vi "ReadFromTxt.vi"(11 "path to PNG file":path) -> (2 "image data":T1)   [LabVIEW 2017]
uses:
  <vilib>/picture/picture.llb/imagedata.ctl
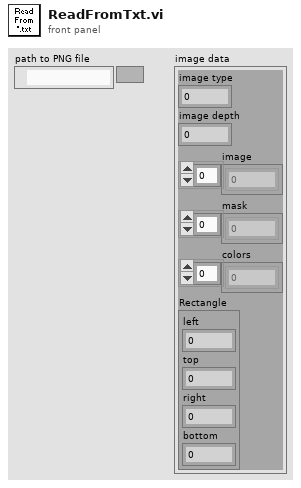
[diagram p1: front panel]
types:
  T1 = typedef "imagedata.ctl" = cluster{"image type":i32, "image depth":i32, "image":u8[], "mask":u8[], "colors":u32[], "Rectangle":cluster{"left":i16, "top":i16, "right":i16, "bottom":i16}}
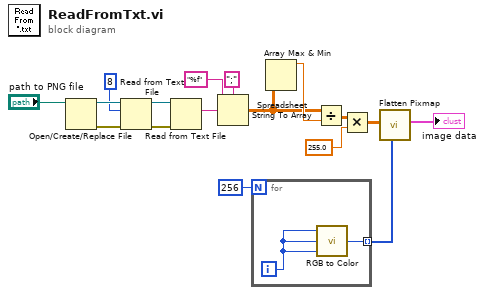
[diagram p0: block diagram]
diagram:
  n1 = Open/Create/Replace File(file path (use dialog)="path to PNG file") -> (refnum out=w9:refnum<file>, error out=w10:errorcluster)  [unwired: 5 in, 1 out]
  n2 = Read from Text File(file (use dialog)=w9, count=8, error in=w10) -> (refnum out=w11:refnum<file>, error out=w12:errorcluster)  [unwired: 1 in, 2 out]
  n3 = Read from Text File(file (use dialog)=w11, error in=w12) -> (text=w13:string)  [unwired: 2 in, 3 out]
  n4 = Spreadsheet String To Array(delimiter (Tab)=";", format string="%f", spreadsheet string=w13) -> (array=w4:dbl[][])  [unwired: 1 in]
  n5 = for {
    N: 256 -> [_]
    tunnel: [w19] -> w1 mode=indexing
    i -> [w18]
    n6 = call <vilib>:"RGB to Color.vi"("B"=w18, "G"=w18, "R"=w18) -> ("Color"=w19:u32)
  }
  n7 = Array Max & Min(array=w4) -> (max value=w5:dbl)  [unwired: 3 out]
  n8 = Divide(x=w4, y=w5) -> (x/y=w6:dbl[][])
  n9 = Multiply(x=w6, y=255.0) -> (x*y=w14:dbl[][])
  n10 = call <vilib>:"Flatten Pixmap.vi"("colors"=w1, "8-bit pixmap"=w14) -> ("image data"=→"image data":T1)  [unwired: 9 in]
